vi "support - acquire data.vi"(8 "error in (no error)":errorcluster) -> (0 "error out":errorcluster, 3 "sin(x)":dbl)   [LabVIEW 2016]
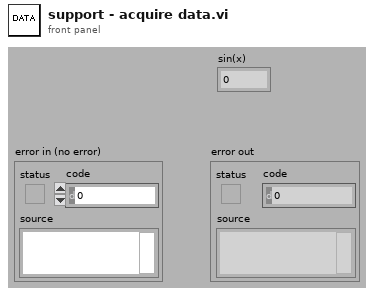
[diagram p1: front panel]
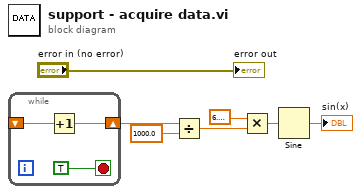
[diagram p0: block diagram]
diagram:
  n1 = while {
    shift-right: [w9] -> w7
    shift-left: _ -> [w10]
    stop <- TRUE stop-if-true
    n2 = Increment(x=w10) -> (x+1=w9:dbl)
  }
  n3 = Divide(x=w7, y=1000.0) -> (x/y=w2:dbl)
  n4 = Multiply(x=6.283185307179586, y=w2) -> (x*y=w1:dbl)
  n5 = Sine(x=w1) -> (sin(x)=→"sin(x)":dbl)
  "error out" <- "error in (no error)"
